vi "Config Steer Module Get-Set.vi"(4 "Start With Default":bool, 6 "Get(f) Set(t)":bool, 7 "Set Steer Values":T1 {"Slot 0 CL"."Gains"."F" format="%#.8f"; "Slot 0 CL"."Gains"."D" format="%#.8f"; "Slot 0 CL"."Gains"."I" format="%#.8f"; "Slot 0 CL"."Gains"."P" format="%#.8f"; "SRX Output"."Min"."REV" format="%.2f"; "SRX Output"."Min"."FWD" format="%.2f"; "SRX Output"."Max"."REV" format="%.2f"; "SRX Output"."Max"."FWD" format="%.2f"}, 8 "Error":errorcluster, 9 "Send Cmd Timout(ms)":u32=300, 11 "Steer Refs":T8) -> (0 "Error Out":errorcluster, 2 "Invert Out":bool, 3 "Steer Refs Out":T8, 5 "Steer Config Out":T1 {"Slot 0 CL"."Gains"."F" format="%#.8f"; "Slot 0 CL"."Gains"."D" format="%#.8f"; "Slot 0 CL"."Gains"."I" format="%#.8f"; "Slot 0 CL"."Gains"."P" format="%#.8f"; "SRX Output"."Min"."REV" format="%.2f"; "SRX Output"."Min"."FWD" format="%.2f"; "SRX Output"."Max"."REV" format="%.2f"; "SRX Output"."Max"."FWD" format="%.2f"})   [LabVIEW 2020, in "Swerve AM_ACT.lvlib"]
uses:
  Swerve AM_ACT.lvlib
  Cluster_Config Steer HW Values.ctl
  Shared Code/TypeDefs/Cluster_Config SRX Motor Output.ctl
  <vilib>/Rock Robotics/WPI/ThirdParty/Phoenix-LabVIEW/Motor Controller/Controls/CTRE_Phoenix_MotorControl_NeutralMode.ctl
  Shared Code/TypeDefs/Cluster_FWD  REV Values.ctl
  Shared Code/TypeDefs/Cluster_SRX SLOT PID Config.ctl
  Shared Code/TypeDefs/Cluster_PID Gains.ctl
  Shared Code/TypeDefs/Cluster_SRX Motion Magic Parameters.ctl
  <vilib>/Rock Robotics/WPI/MotorControl/WPI_MotorControlDeviceRef.ctl
  <vilib>/Rock Robotics/WPI/MotorControl/WPI_MotorControlType.ctl
  <vilib>/Rock Robotics/SystemInterfaces/DIO/FPGA_DIOPWMChannel.ctl
  <vilib>/Rock Robotics/WPI/PWM/WPI_PWMDeadband.ctl
  <vilib>/Rock Robotics/SystemInterfaces/DIO/FPGA_DIOChannel.ctl
  <vilib>/Rock Robotics/WPI/ThirdParty/Phoenix-LabVIEW/Motor Controller/Controls/CTRE_Phoenix_MotorControl_TalonFXMotorControllerConfigurables.ctl
  <vilib>/Rock Robotics/WPI/ThirdParty/Phoenix-LabVIEW/Motor Controller/Controls/CTRE_Phoenix_MotorControl_BaseConfigurables.ctl
  <vilib>/Rock Robotics/WPI/ThirdParty/Phoenix-LabVIEW/Motor Controller/Controls/CTRE_Phoenix_MotorControl_VelocityMeasurementPeriod.ctl
  <vilib>/Rock Robotics/WPI/ThirdParty/Phoenix-LabVIEW/Motor Controller/Controls/CTRE_Phoenix_MotorControl_SlotStructure.ctl
  <vilib>/Rock Robotics/WPI/ThirdParty/Phoenix-LabVIEW/Motor Controller/Controls/CTRE_Phoenix_MotorControl_FilterStruct.ctl
  <vilib>/Rock Robotics/WPI/ThirdParty/Phoenix-LabVIEW/Motor Controller/Controls/CTRE_Phoenix_MotorControl_RemoteSourceType.ctl
  <vilib>/Rock Robotics/WPI/ThirdParty/Phoenix-LabVIEW/Controls/CTRE_Phoenix_CustomParamConfiguration.ctl
  <vilib>/Rock Robotics/WPI/ThirdParty/Phoenix-LabVIEW/Motor Controller/Controls/CTRE_Phoenix_MotorControl_FeedbackDevice_TalonFX.ctl
  <vilib>/Rock Robotics/WPI/ThirdParty/Phoenix-LabVIEW/Motor Controller/Controls/CTRE_Phoenix_MotorControl_LimitSwitchNormal.ctl
  <vilib>/Rock Robotics/WPI/ThirdParty/Phoenix-LabVIEW/Motor Controller/Controls/CTRE_Phoenix_MotorControl_LimitSwitchSource_Local.ctl
  <vilib>/Rock Robotics/WPI/ThirdParty/Phoenix-LabVIEW/Motor Controller/Controls/CTRE_Phoenix_MotorControl_SupplyCurrentLimitConfiguration.ctl
  <vilib>/Rock Robotics/WPI/ThirdParty/Phoenix-LabVIEW/Motor Controller/Controls/CTRE_Phoenix_MotorControl_StatorCurrentLimitConfiguration.ctl
  <vilib>/Rock Robotics/WPI/ThirdParty/Phoenix-LabVIEW/Motor Controller/Controls/CTRE_Phoenix_MotorControl_MotorCommutation_TalonFX.ctl
  <vilib>/Rock Robotics/WPI/ThirdParty/Phoenix-LabVIEW/CANCoder/Controls/CTRE_Phoenix_CANcoder_AbsoluteSensorRange.ctl
  <vilib>/Rock Robotics/WPI/ThirdParty/Phoenix-LabVIEW/CANCoder/Controls/CTRE_Phoenix_CANcoder_SensorInitializationStrategy.ctl
  Shared Code/TypeDefs/Cluser_Config_Current Limits.ctl
  Shared Code/TypeDefs/Cluster_Config_SwerveParam Steer.ctl
  <vilib>/Utility/Data Type/NI_Data Type.lvlib
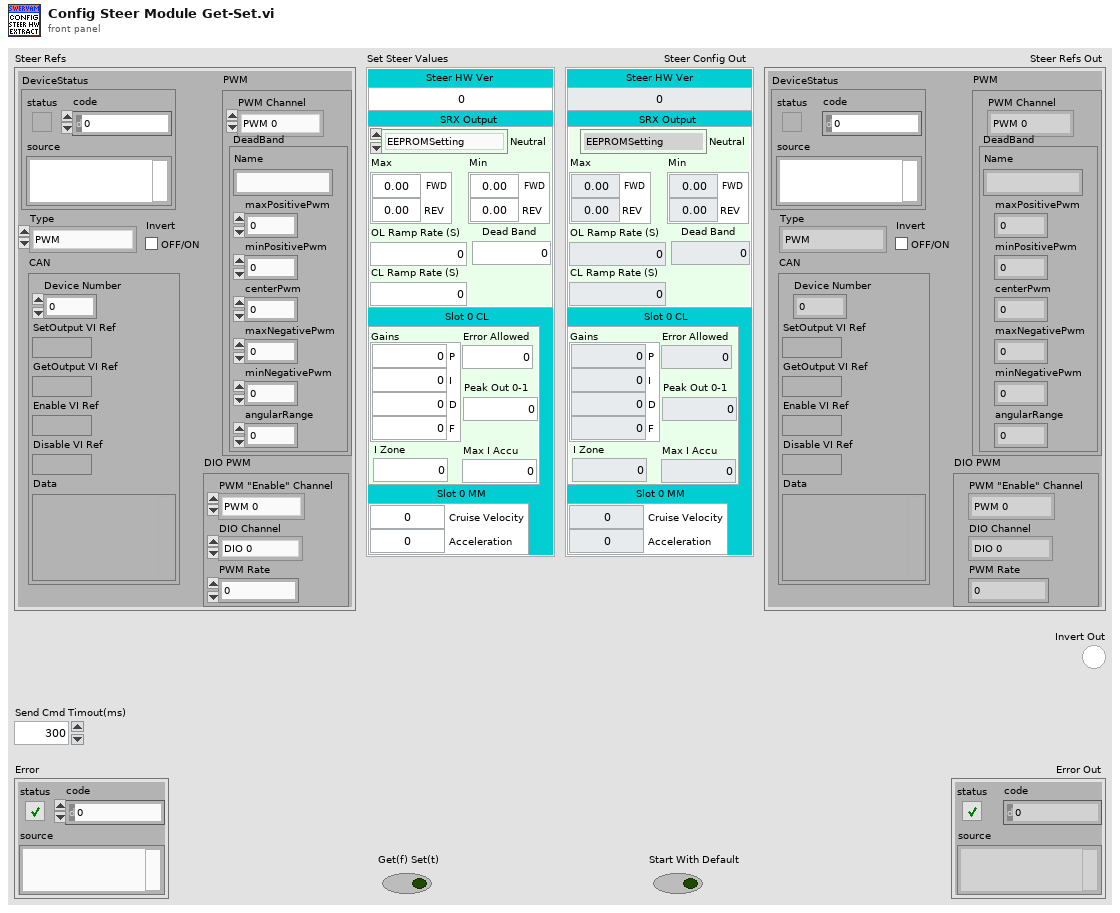
[diagram p1: front panel]
types:
  T1 = typedef "Swerve AM_ACT.lvlib/Cluster_Config Steer HW Values.ctl" = cluster{"Steer HW Ver":u64, "SRX Output":T2, "Slot 0 CL":T5, "Slot 0 MM":T7}
  T2 = typedef "Cluster_Config SRX Motor Output.ctl" = cluster{"Neutral":T3, "Max":T4, "Min":T4, "OL Ramp Rate (S)":dbl, "Dead Band":dbl, "CL Ramp Rate (S)":dbl}
  T3 = typedef "CTRE_Phoenix_MotorControl_NeutralMode.ctl" = enum8{"EEPROMSetting", "Override to Coast", "Override to Brake"}
  T4 = typedef "Cluster_FWD  REV Values.ctl" = cluster{"FWD":dbl, "REV":dbl}
  T5 = typedef "Cluster_SRX SLOT PID Config.ctl" = cluster{"Gains":T6, "Error Allowed":dbl, "I Zone":dbl, "Peak Out 0-1":dbl, "Max I Accu":dbl}
  T6 = typedef "Cluster_PID Gains.ctl" = cluster{"P":dbl, "I":dbl, "D":dbl, "F":dbl}
  T7 = typedef "Cluster_SRX Motion Magic Parameters.ctl" = cluster{"Cruise Velocity":i32, "Acceleration":i32}
  T8 = typedef "WPI_MotorControlDeviceRef.ctl" = cluster{"DeviceStatus":errorcluster, "Type":T9, "PWM":cluster{"PWM Channel":T10, "DeadBand":T11}, "CAN":cluster{"Device Number":u8, "SetOutput VI Ref":variant, "GetOutput VI Ref":variant, "Enable VI Ref":variant, "Disable VI Ref":variant, "Data":variant}, "Invert":bool, "DIO PWM":cluster{"PWM \"Enable\" Channel":T10, "DIOChannel":T12, "PWM Rate":dbl}}
  T9 = typedef "WPI_MotorControlType.ctl" = enum16{"PWM", "CAN", "DIO PWM"}
  T10 = typedef "FPGA_DIOPWMChannel.ctl" = enum8{"PWM 0", "PWM 1", "PWM 2", "PWM 3", "PWM 4", "PWM 5", "PWM 6", "PWM 7", "PWM 8", "PWM 9", "PWM MXP 0", "PWM MXP 1", "PWM MXP 2", "PWM MXP 3", "PWM MXP 4", "PWM MXP 5", "PWM MXP 6", "PWM MXP 7", "PWM MXP 8", "PWM MXP 9", "Invalid"}
  T11 = typedef "WPI_PWMDeadband.ctl" = cluster{"Name":string, "maxPositivePwm":i32, "minPositivePwm":i32, "centerPwm":i32, "maxNegativePwm":i32, "minNegativePwm":i32, "angularRange":u16}
  T12 = typedef "FPGA_DIOChannel.ctl" = enum8{"DIO 0", "DIO 1", "DIO 2", "DIO 3", "DIO 4", "DIO 5", "DIO 6", "DIO 7", "DIO 8", "DIO 9", "DIO MXP 0", "DIO MXP 1", "DIO MXP 2", "DIO MXP 3", "DIO MXP 4", "DIO MXP 5", "DIO MXP 6", "DIO MXP 7", "DIO MXP 8", "DIO MXP 9", "DIO MXP 10", "DIO MXP 11", "DIO MXP 12", "DIO MXP 13", "DIO MXP 14", "DIO MXP 15", "SPI Port CS1", "SPI Port CS2", "SPI Port CS3", "SPI Port MISO", "SPI Port MOSI", "Invalid"}
  T13 = typedef "CTRE_Phoenix_MotorControl_TalonFXMotorControllerConfigurables.ctl" = cluster{"Base Configurables":T14, "primaryPID":cluster{"selectedFeedbackCoefficient":dbl, "selectedFeedbackSensor":T20}, "auxiliaryPID":cluster{"selectedFeedbackCoefficient":dbl, "selectedFeedbackSensor":T20}, "forwardLimitSwitchNormal":T21, "reverseLimitSwitchNormal":T21, "forwardLimitSwitchDeviceID":i32, "reverseLimitSwitchDeviceID":i32, "forwardLimitSwitchSource":T22, "reverseLimitSwitchSource":T22, "sum0Term":T20, "sum1Term":T20, "diff0Term":T20, "diff1Term":T20, "Supply Current Limit Configuration":T23, "Stator Current Limit Configuration":T24, "Motor Commutation":T25, "Absolute Sensor Range":T26, "Integrated Sensor Offset (Degrees)":dbl, "Sensor Initialization Strategy":T27}
  T14 = typedef "CTRE_Phoenix_MotorControl_BaseConfigurables.ctl" = cluster{"openLoopRamp":dbl, "closedLoopRamp":dbl, "peakOutputForward":dbl, "peakOutputReverse":dbl, "nominalOutputForward":dbl, "nominalOutputReverse":dbl, "neutralDeadband":dbl, "voltageCompSaturation":dbl, "voltageMeasurementFilter":i32, "velocityMeasurementPeriod":T15, "velocityMeasurementWindow":i32, "forwardSoftLimitThreshold":i32, "reverseSoftLimitThreshold":i32, "forwardSoftLimitEnable":bool, "reverseSoftLimitEnable":bool, "slot0":T16, "slot1":T16, "slot2":T16, "slot3":T16, "auxPIDPolarity":bool, "remoteFilter0":T17, "remoteFilter1":T17, "motionCruiseVelocity":i32, "motionAcceleration":i32, "motionProfileTrajectoryPeriod":i32, "feedbackNotContinuous":bool, "remoteSensorClosedLoopDisableNeutralOnLOS":bool, "clearPositionOnLimitF":bool, "clearPositionOnLimitR":bool, "clearPositionOnQuadIdx":bool, "limitSwitchDisableNeutralOnLOS":bool, "softLimitDisableNeutralOnLOS":bool, "pulseWidthPeriod_EdgesPerRot":i32, "pulseWidthPeriod_FilterWindowSz":i32, "customParam":T19, "trajectoryInterpolationEnable":bool}
  T15 = typedef "CTRE_Phoenix_MotorControl_VelocityMeasurementPeriod.ctl" = u16
  T16 = typedef "CTRE_Phoenix_MotorControl_SlotStructure.ctl" = cluster{"P":dbl, "I":dbl, "D":dbl, "F":dbl, "integralZone":dbl, "allowableClosedLoopError":i32, "maxIntegralAccumulator":dbl, "closedLoopPeakOutput":dbl, "closedLoopPeriod":i32}
  T17 = typedef "CTRE_Phoenix_MotorControl_FilterStruct.ctl" = cluster{"remoteSensorDeviceID":u8, "remoteSensorSource":T18}
  T18 = typedef "CTRE_Phoenix_MotorControl_RemoteSourceType.ctl" = enum16{"Off", "Talon SRX Selected Sensor", "Pigeon IMU Yaw", "Pigeon IMU Pitch", "Pigeon IMU Roll", "CANifier Quadrature", "CANifier PWM Input 0", "CANifier PWM Input 1", "CANifier PWM Input 2", "CANifier PWM Input 3", "Gadgeteer Pigeon Yaw", "Gadgeteer Pigeon Pitch", "Gadgeteer Pigeon Roll", "CANCoder"}
  T19 = typedef "CTRE_Phoenix_CustomParamConfiguration.ctl" = cluster{"customParam0":i32, "customParam1":i32}
  T20 = typedef "CTRE_Phoenix_MotorControl_FeedbackDevice_TalonFX.ctl" = i8
  T21 = typedef "CTRE_Phoenix_MotorControl_LimitSwitchNormal.ctl" = enum16{"Normally Open", "Normally Closed", "Disabled"}
  T22 = typedef "CTRE_Phoenix_MotorControl_LimitSwitchSource_Local.ctl" = enum16{"Feedback Connector", "Remote Talon SRX", "Remote CANifier", "Deactivated"}
  T23 = typedef "CTRE_Phoenix_MotorControl_SupplyCurrentLimitConfiguration.ctl" = cluster{"Enable?":bool, "Current Limit":dbl, "Threshold Current":dbl, "Threshold Time":dbl}
  T24 = typedef "CTRE_Phoenix_MotorControl_StatorCurrentLimitConfiguration.ctl" = cluster{"Enable?":bool, "Current Limit":dbl, "Threshold Current":dbl, "Threshold Time":dbl}
  T25 = typedef "CTRE_Phoenix_MotorControl_MotorCommutation_TalonFX.ctl" = enum16{"Trapezoidal"}
  T26 = typedef "CTRE_Phoenix_CANcoder_AbsoluteSensorRange.ctl" = enum16{"Unsigned [0 to 360)", "Signed [-180 to +180)"}
  T27 = typedef "CTRE_Phoenix_CANcoder_SensorInitializationStrategy.ctl" = enum16{"Boot To Zero", "Boot To Absolute Position"}
  T28 = typedef "Cluster_Config_SwerveParam Steer.ctl" = cluster{"CPR":dbl}
  T29 = typedef "Cluser_Config_Current Limits.ctl" = cluster{"Enable":bool, "Current Limit":dbl, "Threshold Current":dbl, "Threshold Time":dbl}
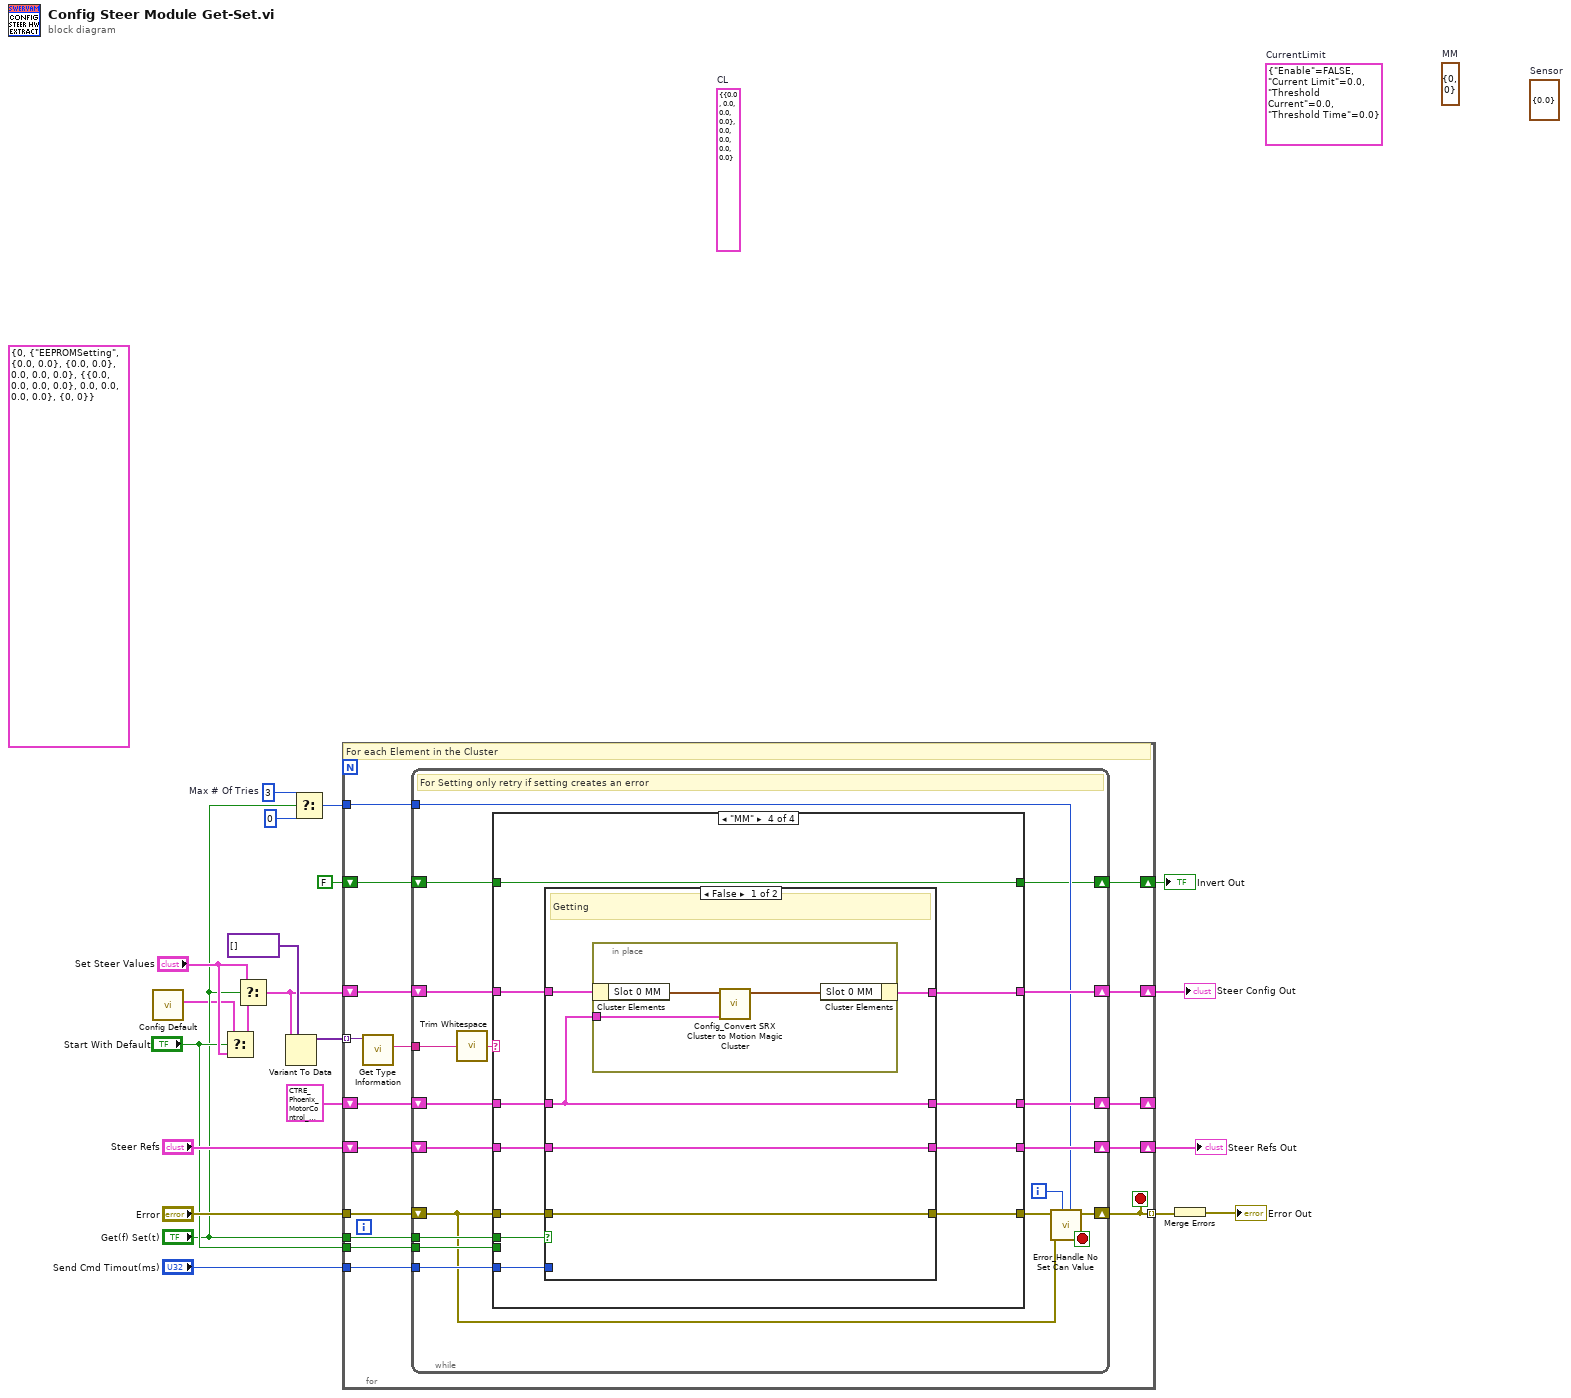
[diagram p0: block diagram]
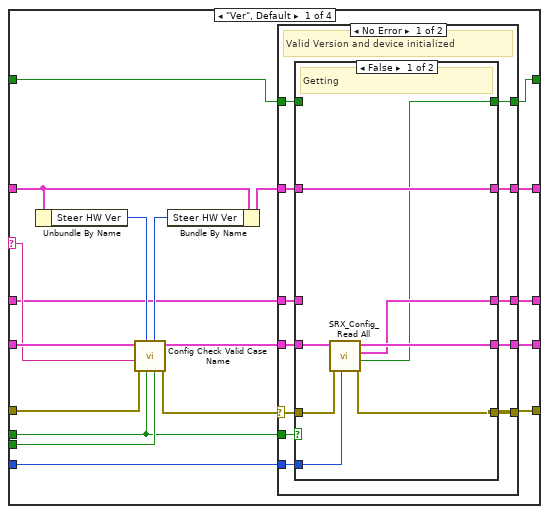
[diagram p2: hidden frame]
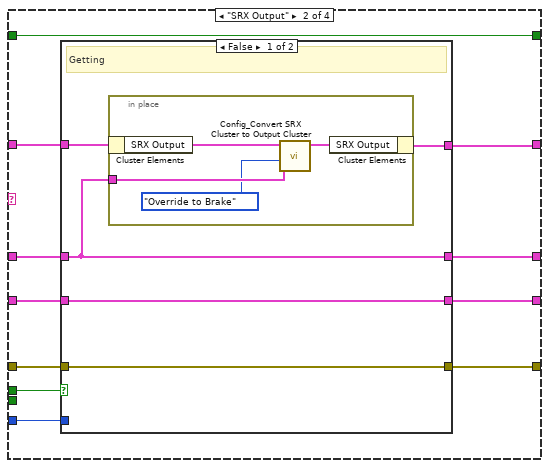
[diagram p5: hidden frame]
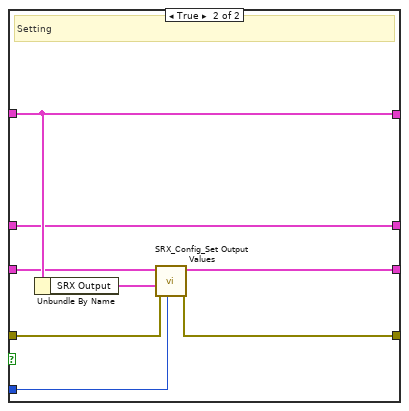
[diagram p6: hidden frame]
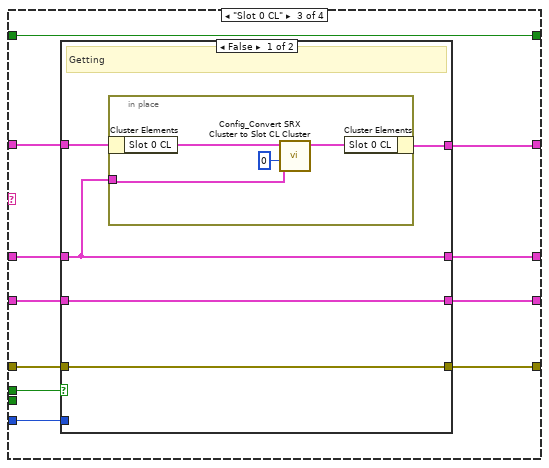
[diagram p7: hidden frame]
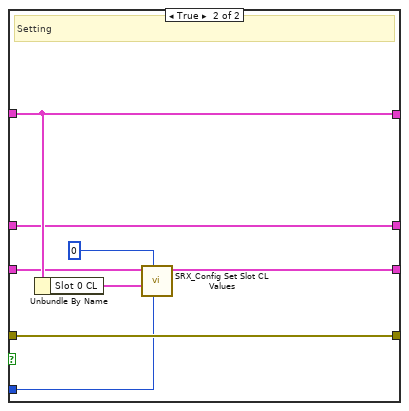
[diagram p8: hidden frame]
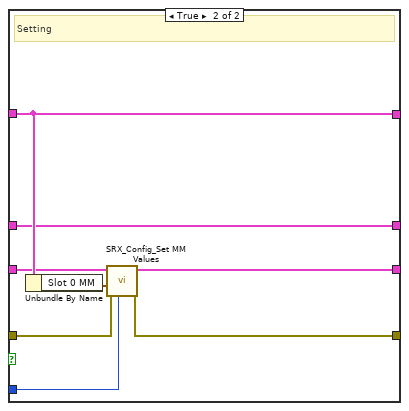
[diagram p9: hidden frame]
diagram:
  w5 = 3  # Max # Of Tries
  (unwired) T1 {"Steer HW Ver"=0, "SRX Output"={"Neutral"=enum."EEPROMSetting", "Max"={"FWD"=0.0, "REV"=0.0}, "Min"={"FWD"=0.0, "REV"=0.0}, "OL Ramp Rate (S)"=0.0, "Dead Band"=0.0, "CL Ramp Rate (S)"=0.0}, "Slot 0 CL"={"Gains"={"P"=0.0, "I"=0.0, "D"=0.0, "F"=0.0}, "Error Allowed"=0.0, "I Zone"=0.0, "Peak Out 0-1"=0.0, "Max I Accu"=0.0}, "Slot 0 MM"={"Cruise Velocity"=0, "Acceleration"=0}} ("Set Steer Values")
  (unwired) T28 {"CPR"=0.0}  # Sensor
  (unwired) T7 {"Cruise Velocity"=0, "Acceleration"=0}  # MM
  (unwired) T29 {"Enable"=FALSE, "Current Limit"=0.0, "Threshold Current"=0.0, "Threshold Time"=0.0}  # CurrentLimit
  (unwired) T5 {"Gains"={"P"=0.0, "I"=0.0, "D"=0.0, "F"=0.0}, "Error Allowed"=0.0, "I Zone"=0.0, "Peak Out 0-1"=0.0, "Max I Accu"=0.0}  # CL
  n1 = call "Config Default.vi"() -> ("Steer Default Out"=w3:T1)  [unwired: 8 in, 3 out]
  n2 = Select(t=w3, s="Start With Default", f="Set Steer Values") -> (s? t:f=w11:T1)
  n3 = Select(t="Set Steer Values", s="Get(f) Set(t)", f=w11) -> (s? t:f=w13:T1)
  n4 = Variant To Data(type=variant[] [], Variant=w13) -> (data=w19:variant[])  [unwired: 1 in, 1 out]
  n5 = Select(t=w5, s="Get(f) Set(t)", f=0) -> (s? t:f=w4:i32)
  n6 = for {
    tunnel: w19 -> [w36] mode=indexing
    shift-right: [w33] -> w18
    shift-left: w13 -> [w34]
    tunnel: "Error" -> [w32]
    tunnel: [w31] -> w17 mode=indexing
    shift-right: [w30] -> w14
    shift-left: "Steer Refs" -> [w35]
    tunnel: "Get(f) Set(t)" -> [w29]
    tunnel: "Start With Default" -> [w28]
    shift-right: [w26] -> _
    shift-left: T13 {"Base Configurables"={"openLoopRamp"=0.0, "closedLoopRamp"=0.0, "peakOutputForward"=0.0, "peakOutputReverse"=0.0, "nominalOutputForward"=0.0, "nominalOutputReverse"=0.0, "neutralDeadband"=0.0, "voltageCompSaturation"=0.0, "voltageMeasurementFilter"=0, "velocityMeasurementPeriod"=0, "velocityMeasurementWindow"=0, "forwardSoftLimitThreshold"=0, "reverseSoftLimitThreshold"=0, "forwardSoftLimitEnable"=FALSE, "reverseSoftLimitEnable"=FALSE, "slot0"={"P"=0.0, "I"=0.0, "D"=0.0, "F"=0.0, "integralZone"=0.0, "allowableClosedLoopError"=0, "maxIntegralAccumulator"=0.0, "closedLoopPeakOutput"=0.0, "closedLoopPeriod"=0}, "slot1"={"P"=0.0, "I"=0.0, "D"=0.0, "F"=0.0, "integralZone"=0.0, "allowableClosedLoopError"=0, "maxIntegralAccumulator"=0.0, "closedLoopPeakOutput"=0.0, "closedLoopPeriod"=0}, "slot2"={"P"=0.0, "I"=0.0, "D"=0.0, "F"=0.0, "integralZone"=0.0, "allowableClosedLoopError"=0, "maxIntegralAccumulator"=0.0, "closedLoopPeakOutput"=0.0, "closedLoopPeriod"=0}, "slot3"={"P"=0.0, "I"=0.0, "D"=0.0, "F"=0.0, "integralZone"=0.0, "allowableClosedLoopError"=0, "maxIntegralAccumulator"=0.0, "closedLoopPeakOutput"=0.0, "closedLoopPeriod"=0}, "auxPIDPolarity"=FALSE, "remoteFilter0"={"remoteSensorDeviceID"=0, "remoteSensorSource"=enum."Off"}, "remoteFilter1"={"remoteSensorDeviceID"=0, "remoteSensorSource"=enum."Off"}, "motionCruiseVelocity"=0, "motionAcceleration"=0, "motionProfileTrajectoryPeriod"=0, "feedbackNotContinuous"=FALSE, "remoteSensorClosedLoopDisableNeutralOnLOS"=FALSE, "clearPositionOnLimitF"=FALSE, "clearPositionOnLimitR"=FALSE, "clearPositionOnQuadIdx"=FALSE, "limitSwitchDisableNeutralOnLOS"=FALSE, "softLimitDisableNeutralOnLOS"=FALSE, "pulseWidthPeriod_EdgesPerRot"=0, "pulseWidthPeriod_FilterWindowSz"=0, "customParam"={"customParam0"=0, "customParam1"=0}, "trajectoryInterpolationEnable"=FALSE}, "primaryPID"={"selectedFeedbackCoefficient"=0.0, "selectedFeedbackSensor"=0}, "auxiliaryPID"={"selectedFeedbackCoefficient"=0.0, "selectedFeedbackSensor"=0}, "forwardLimitSwitchNormal"=enum."Normally Open", "reverseLimitSwitchNormal"=enum."Normally Open", "forwardLimitSwitchDeviceID"=0, "reverseLimitSwitchDeviceID"=0, "forwardLimitSwitchSource"=enum."Feedback Connector", "reverseLimitSwitchSource"=enum."Feedback Connector", "sum0Term"=0, "sum1Term"=0, "diff0Term"=0, "diff1Term"=0, "Supply Current Limit Configuration"={"Enable?"=FALSE, "Current Limit"=0.0, "Threshold Current"=0.0, "Threshold Time"=0.0}, "Stator Current Limit Configuration"={"Enable?"=FALSE, "Current Limit"=0.0, "Threshold Current"=0.0, "Threshold Time"=0.0}, "Motor Commutation"=enum."Trapezoidal", "Absolute Sensor Range"=enum."Unsigned [0 to 360)", "Integrated Sensor Offset (Degrees)"=0.0, "Sensor Initialization Strategy"=enum."Boot To Zero"} ("FX Config Out") -> [w25]
    tunnel: "Send Cmd Timout(ms)" -> [w27]
    tunnel: w4 -> [w24]
    shift-right: [w22] -> w1
    shift-left: FALSE -> [w23]
    stop <- w31 stop-if-true
    # "For each Element in the Cluster"
    n7 = call <vilib>:"Get Type Information.vi"("variant"=w36) -> ("name"=w37:string)  [unwired: 6 in, 4 out]
    n8 = while {
      tunnel: w37 -> [w56]
      tunnel: w29 -> [w50]
      tunnel: w28 -> [w49]
      tunnel: w27 -> [w48]
      shift-right: [w51] -> w30
      shift-left: w35 -> [w54]
      shift-right: [w52] -> w33
      shift-left: w34 -> [w53]
      shift-right: [w43] -> w31
      shift-left: w32 -> [w45]
      shift-right: [w47] -> w26
      shift-left: w25 -> [w46]
      tunnel: w24 -> [w40]
      shift-right: [w38] -> w22
      shift-left: w23 -> [w39]
      i -> [w41]
      stop <- w42 stop-if-true
      # "For Setting only retry if setting creates an error"
      n9 = call <vilib>:"Trim Whitespace.vi"("string"=w56) -> ("trimmed string"=w55:string)  [unwired: 1 in]
      n10 = case shown="\"MM\"" w55 {
        selector: w55 -> [w69 _ _ _]
        tunnel: w54 -> [w72 w112 w140 w168]
        tunnel: w53 -> [w70 w116 w144 w172]
        tunnel: [w62 w115 w143 w171] -> w52
        tunnel: w45 -> [w75 w111 w139 w167]
        tunnel: [w67 w109 w137 w165] -> w44
        tunnel: [w65 w110 w138 w166] -> w51
        tunnel: w50 -> [w60 w113 w141 w169]
        tunnel: w49 -> [w71 _ _ _]
        tunnel: w48 -> [w64 w107 w135 w163]
        tunnel: [w63 w108 w136 w164] -> w47
        tunnel: w46 -> [w59 w114 w142 w170]
        tunnel: w39 -> [w58 w106 w134 w162]
        tunnel: [w57 w106 w134 w162] -> w38
        frame "Ver", Default {
          n11 = Unbundle By Name(w70) -> ("Steer HW Ver"=w74:u64)
          n12 = call "Config Check Valid Case Name.vi"("Start With Default"=w71, "Get(f) Set(t)"=w60, "Ver"=w74, "Error"=w75, "Case Name"=w69, "Steer Refs"=w72) -> ("Error Out"=w68:errorcluster, "Steer Refs Out"=w66:T8, "Ver Out"=w73:u64)  [unwired: 3 in]
          n13 = Bundle By Name(cluster=w70, "Steer HW Ver"=w73) -> (w61:T1)
          n14 = case shown="No Error" w68 {
            selector: w68 -> [w87 w104]
            tunnel: [w86 w104] -> w67
            tunnel: w66 -> [w85 w105]
            tunnel: [w84 w105] -> w65
            tunnel: w64 -> [w83 _]
            tunnel: [w82 w102] -> w63
            tunnel: [w81 w103] -> w62
            tunnel: w61 -> [w80 w103]
            tunnel: w60 -> [w79 _]
            tunnel: w59 -> [w78 w102]
            tunnel: w58 -> [w77 w101]
            tunnel: [w76 w101] -> w57
            frame No Error {
              # "Valid Version and device initialized"
              n15 = case shown="False" w79 {
                tunnel: w87 -> [w95 w97]
                tunnel: [w94 w97] -> w86
                tunnel: w85 -> [w93 w99]
                tunnel: [w92 w99] -> w84
                tunnel: w83 -> [w91 _]
                tunnel: [w90 w98] -> w82
                tunnel: [w89 w100] -> w81
                tunnel: w80 -> [w89 w100]
                tunnel: w78 -> [_ w98]
                tunnel: w77 -> [_ w96]
                tunnel: [w88 w96] -> w76
                frame False {
                  # "Getting"
                  n16 = call "SRX_Config_Read All.vi"("Send Cmd Timout(ms)"=w91, "Error"=w95, "PhoenixMotorControlDevRef"=w93) -> ("Error Out"=w94:errorcluster, "Inverted? Out"=w88:bool, "FX Config Out"=w90:T13, "Ref Out"=w92:T8)  [unwired: 5 in]
                }
                frame True {
                  # "Setting"
                }
              }
            }
            frame Error {
            }
          }
        }
        frame "SRX Output" {
          n17 = case shown="False" w113 {
            tunnel: w116 -> [w121 w133]
            tunnel: [w120 w133] -> w115
            tunnel: w114 -> [w117 w132]
            tunnel: w112 -> [w119 w129]
            tunnel: w111 -> [w118 w126]
            tunnel: [w119 w130] -> w110
            tunnel: [w118 w127] -> w109
            tunnel: [w117 w132] -> w108
            tunnel: w107 -> [_ w128]
            frame False {
              # "Getting"
              n18 = in-place {
                in-place-border: w117 -> [w125]
                n19 = in-place-cluster #1(w121) -> ("SRX Output"=w124:T2)
                n20 = call "Config_Convert SRX Cluster to Output Cluster.vi"("SRX Config"=w125, "Neutral Mode"=CTRE_Phoenix_MotorControl_NeutralMode."Override to Brake", "SRX Output"=w124) -> ("SRX Output Out"=w123:T2)  [unwired: 8 in]
                n21 = in-place-cluster #1("SRX Output"=w123) -> (w120:T1)
              }
            }
            frame True {
              # "Setting"
              n22 = Unbundle By Name(w133) -> ("SRX Output"=w131:T2)
              n23 = call "SRX_Config_Set Output Values.vi"("Send Cmd Timout(ms)"=w128, "Error"=w126, "SRX Output"=w131, "PhoenixMotorControlDevRef"=w129) -> ("Error Out"=w127:errorcluster, "PhoenixMotorControlDevRef Out"=w130:T8)  [unwired: 6 in]
            }
          }
        }
        frame "Slot 0 CL" {
          n24 = case shown="False" w141 {
            tunnel: w144 -> [w149 w161]
            tunnel: [w148 w161] -> w143
            tunnel: w142 -> [w145 w160]
            tunnel: w140 -> [w147 w157]
            tunnel: w139 -> [w146 w159]
            tunnel: [w147 w158] -> w138
            tunnel: [w146 w159] -> w137
            tunnel: [w145 w160] -> w136
            tunnel: w135 -> [_ w156]
            frame False {
              # "Getting"
              n25 = in-place {
                in-place-border: w145 -> [w150]
                n26 = in-place-cluster #2(w149) -> ("Slot 0 CL"=w151:T5)
                n27 = call "Config_Convert SRX Cluster to Slot CL Cluster.vi"("SRX Config Out"=w150, "Slot"=0, "Slot 0 CL"=w151) -> ("Slot 0 CL Out"=w153:T5)  [unwired: 7 in, 1 out]
                n28 = in-place-cluster #2("Slot 0 CL"=w153) -> (w148:T1)
              }
            }
            frame True {
              # "Setting"
              n29 = Unbundle By Name(w161) -> ("Slot 0 CL"=w154:T5)
              n30 = call "SRX_Config Set Slot CL Values.vi"("Send Cmd Timout(ms)"=w156, "SlotIdx"=0, "CL"=w154, "PhoenixMotorControlDevRef"=w157) -> ("PhoenixMotorControlDevRef Out"=w158:T8)  [unwired: 5 in, 2 out]
            }
          }
        }
        frame "MM" {
          n31 = case shown="False" w169 {
            tunnel: w172 -> [w177 w188]
            tunnel: [w176 w188] -> w171
            tunnel: w170 -> [w173 w187]
            tunnel: w168 -> [w175 w185]
            tunnel: w167 -> [w174 w183]
            tunnel: [w175 w186] -> w166
            tunnel: [w174 w184] -> w165
            tunnel: [w173 w187] -> w164
            tunnel: w163 -> [_ w182]
            frame False {
              # "Getting"
              n32 = in-place {
                in-place-border: w173 -> [w178]
                n33 = in-place-cluster #3(w177) -> ("Slot 0 MM"=w180:T7)
                n34 = call "Config_Convert SRX Cluster to Motion Magic Cluster.vi"("SRX Config"=w178, "MM"=w180) -> ("Output Cluster Out"=w179:T7)  [unwired: 9 in]
                n35 = in-place-cluster #3("Slot 0 MM"=w179) -> (w176:T1)
              }
            }
            frame True {
              # "Setting"
              n36 = Unbundle By Name(w188) -> ("Slot 0 MM"=w181:T7)
              n37 = call "SRX_Config_Set MM Values.vi"("Send Cmd Timout(ms)"=w182, "Error"=w183, "MM"=w181, "PhoenixMotorControlDevRef"=w185) -> ("Error Out"=w184:errorcluster, "PhoenixMotorControlDevRef Out"=w186:T8)  [unwired: 6 in]
            }
          }
        }
      }
      n38 = call "Error_Handle No Set Can Value.vi"("Max # Of Tries"=w40, "Loop Itteration"=w41, "Previous Error"=w45, "Error"=w44) -> ("Stop Out"=w42:bool, "Error Out"=w43:errorcluster)  [unwired: 6 in]
    }
  }
  "Steer Refs Out" <- w14
  "Steer Config Out" <- w18
  "Invert Out" <- w1
  n39 = Merge Errors(w17) -> (→"Error Out":errorcluster)
